vi "Arduino(test).vi"() -> ()   [LabVIEW 2014]
uses:
  <vilib>/MakerHub/LINX/Public/Peripherals/Digital/Digital Write 1 Chan.vi
  <vilib>/MakerHub/LINX/Public/Peripherals/Analog/Analog Read N Chans.vi
  <vilib>/MakerHub/LINX/Public/Peripherals/Digital/Digital Write N Chans.vi
  <vilib>/MakerHub/LINX/Private/Local IO/LinxAnalogRead.vi
  <vilib>/MakerHub/LINX/Public/Utilities/Check Channel.vi
  <vilib>/MakerHub/LINX/Private/Local IO/LinxDigitalWrite.vi
  <vilib>/MakerHub/LINX/Public/Utilities/Open Serial.vi
  <vilib>/MakerHub/LINX/Private/Utilties/Generate Error.vi
  <vilib>/MakerHub/LINX/LMH-LINX.lvlib
panel:
  out "cluster":T1
  out "Heating W":bool
  in  "Pump":bool
  out "Pump":bool
  out "Pressure, mm Hg":dbl(knob) scale=700.0..780.0
  out "Temp Whater":dbl(slide) scale=10.0..40.0 scale format="%#.1g"
  out "Tank, l":dbl(slide) scale=0.0..50.0 scale format="%#.1g"
  out "Lighting":bool
  out "Lighting, Klm":dbl(knob) scale=0.0..28.0
  out "Time":timestamp format="%<%H:%M:%S\n%d/%m/%y>T"
  out "Heating":bool
  out "Watering":bool
  out "Dry":bool
  out "Humidity, %":dbl(knob) scale=0.0..100.0
  out "Temp Air":dbl(slide) scale=10.0..40.0 scale format="%#.1g"
  in  "stop":bool
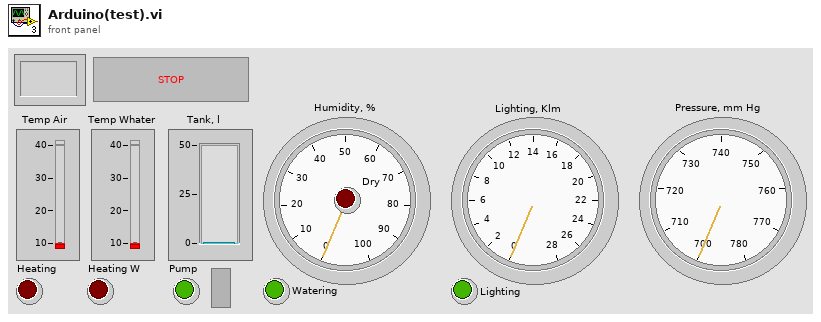
[diagram p1: front panel]
types:
  T1 = cluster{"Voltages[0]":dbl, "Voltages[1]":dbl, "Voltages[2]":dbl, "Voltages[3]":dbl, "Voltages[4]":dbl, "Voltages[5]":dbl, "Voltages[6]":dbl, "Voltages[7]":dbl, "Voltages[8]":dbl}
  T2 = typedef "LMH-LINX.lvlib/LINX Ref.ctl" = cluster{"IO":T3, "Interface":T4, "LINX Device Config":T5}
  T3 = typedef "LMH-LINX.lvlib/Platform.ctl" = enum16{"Remote", "Local"}
  T4 = typedef "LMH-LINX.lvlib/Interface.ctl" = enum16{"Serial", "TCP"}
  T5 = typedef "LMH-LINX.lvlib/Device.lvlib/LINX Device Config.ctl" = cluster{"Interface":T4, "COM Port":refnum<visa-resource-name>, "TCP Configuration":T6, "Device Family":u8, "Device ID":u8, "Device Name":string, "TCP Ref":refnum<k5>, "Channels":T7}
  T6 = typedef "LMH-LINX.lvlib/Device.lvlib/TCP Config.ctl" = cluster{"IP Address":string, "Port":u16}
  T7 = typedef "LMH-LINX.lvlib/Channels.ctl" = cluster{"DI":u8[], "DO":u8[], "AI":u8[], "AO":u8[], "PWM":u8[], "QE":u8[], "UART":u8[], "I2C 2":u8[], "SPI":u8[], "CAN":u8[], "Servo":u8[], "AI Ref (V)":dbl, "AI Resolution (Bits)":u8, "AO Ref (V)":dbl, "AO Resolution (Bits)":u8}
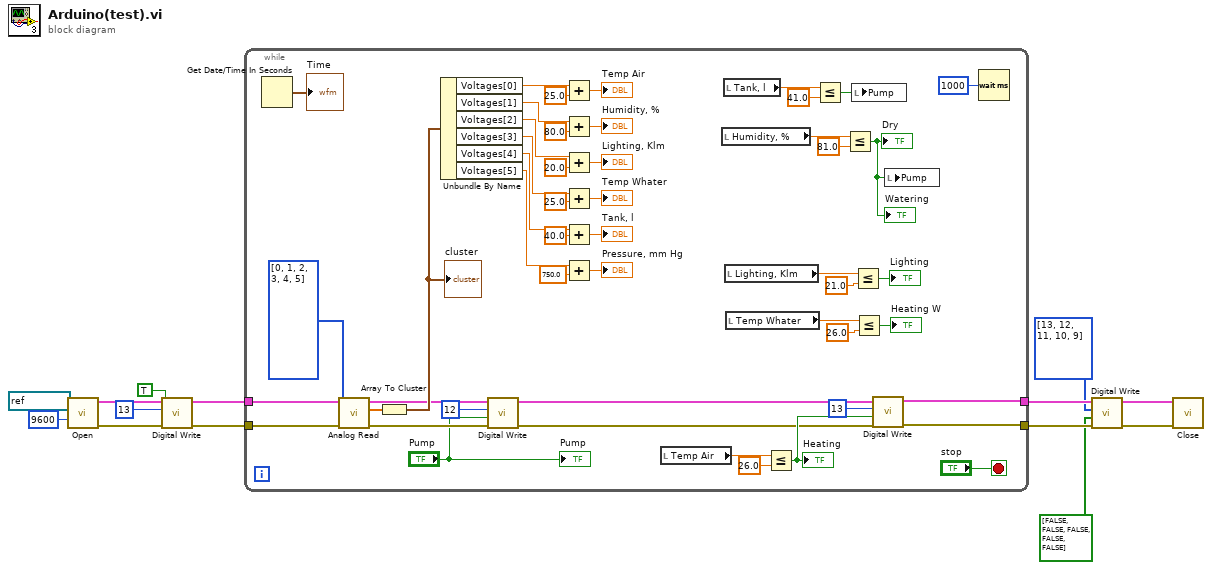
[diagram p0: block diagram]
diagram:
  n1 = call-poly <vilib>:"Open.vi"("Baud Rate Override"=u32 9600, "Serial Port"=refnum<visa-resource-name> "COM4") -> ("Error Out"=w11:errorcluster, "LINX Resource"=w12:T2)  [unwired: 7 in, 1 out]
  n2 = call-poly <vilib>:"Digital Write.vi"("Error In"=w11, "Output Value"=TRUE, "DO Channel"=u8 13, "LINX Resource"=w12) -> ("Error Out"=w9:errorcluster, "LINX Resource"=w10:T2)  [unwired: 6 in]
  n3 = while {
    tunnel: w10 -> [w62]
    tunnel: w9 -> [w63]
    tunnel: [w33] -> w6
    tunnel: [w32] -> w5
    stop <- "stop" stop-if-true
    n4 = Get Date/Time In Seconds() -> (seconds since 1Jan1904=→"Time":timestamp)
    n5 = call-poly <vilib>:"Analog Read.vi"("Error In"=w63, "AI Channel(s)"=u8[] [0, 1, 2, 3, 4, 5], "LINX Resource"=w62) -> ("Error Out"=w38:errorcluster, "Voltages"=w59:dbl[], "LINX Resource"=w39:T2)  [unwired: 5 in, 1 out]
    n6 = Array To Cluster(array=w59) -> (cluster=w58:T1)
    "cluster" <- w58
    n7 = Unbundle By Name(w58) -> ("Voltages[0]"=w55:dbl, "Voltages[1]"=w52:dbl, "Voltages[2]"=w50:dbl, "Voltages[3]"=w41:dbl, "Voltages[4]"=w17:dbl, "Voltages[5]"=w40:dbl)
    n8 = call-poly <vilib>:"Digital Write.vi"("Error In"=w38, "Output Value"="Pump", "DO Channel"=u8 12, "LINX Resource"=w39) -> ("Error Out"=w15:errorcluster, "LINX Resource"=w16:T2)  [unwired: 6 in]
    n9 = Add(x=w55, y=25.0) -> (x+y=→"Temp Air":dbl)
    n10 = Add(x=w52, y=80.0) -> (x+y=→"Humidity, %":dbl)
    n11 = Add(x=w50, y=20.0) -> (x+y=→"Lighting, Klm":dbl)
    n12 = Add(x=w41, y=25.0) -> (x+y=→"Temp Whater":dbl)
    n13 = Add(x=w17, y=40.0) -> (x+y=→"Tank, l":dbl)
    n14 = Add(x=w40, y=750.0) -> (x+y=→"Pressure, mm Hg":dbl)
    n15 = local read "Temp Air"() -> (w35:dbl)
    n16 = local read "Humidity, %"() -> (w26:dbl)
    n17 = local read "Tank, l"() -> (w29:dbl)
    n18 = local read "Lighting, Klm"() -> (w20:dbl)
    n19 = local read "Temp Whater"() -> (w21:dbl)
    n20 = Less Or Equal?(x=w35, y=26.0) -> (x <= y?=w31:bool)
    "Heating" <- w31
    n21 = Less Or Equal?(x=w29, y=41.0) -> (x <= y?=w28:bool)
    n22 = Less Or Equal?(x=w26, y=81.0) -> (x <= y?=w24:bool)
    "Dry" <- w24
    "Watering" <- w24
    n23 = local write "Pump"(w28) -> ()
    n24 = Less Or Equal?(x=w20, y=21.0) -> (x <= y?=→"Lighting":bool)
    n25 = Less Or Equal?(x=w21, y=26.0) -> (x <= y?=→"Heating W":bool)
    n26 = call-poly <vilib>:"Digital Write.vi"("Error In"=w15, "Output Value"=w31, "DO Channel"=u8 13, "LINX Resource"=w16) -> ("Error Out"=w32:errorcluster, "LINX Resource"=w33:T2)  [unwired: 6 in]
    n27 = local write "Pump"(w24) -> ()
    n28 = Wait (ms)(milliseconds to wait=u32 1000) -> ()  [unwired: 1 out]
    "Pump" <- "Pump"
  }
  n29 = call-poly <vilib>:"Digital Write.vi"("Error In"=w5, "Values"=bool[] [FALSE, FALSE, FALSE, FALSE, FALSE], "DO Channels"=u8[] [13, 12, 11, 10, 9], "LINX Resource"=w6) -> ("Error Out"=w3:errorcluster, "LINX Resource"=w4:T2)  [unwired: 6 in]
  n30 = call <vilib>:"Close.vi"("Error In"=w3, "LINX Resource"=w4) -> ()  [unwired: 9 in, 1 out]
